vi "DVR Read - CAN Configuration.vi"(11 "Data Value Reference in":refnum<data-value>) -> (3 "CAN Port Configuration":T1 {"Sample Rate (Hz)" format="%#_13g"})   [LabVIEW 2021, in "Performanced XNET CAN Signal Logger.lvlib" / "Performanced XNET CAN Signal Logger.lvclass"]
uses:
  Performanced XNET CAN Signal Logger.lvclass
  Typedef/Def-CAN Port Configuration.ctl
  Performanced XNET CAN Signal Logger.lvclass/Performanced XNET CAN Signal Logger.ctl
  XNET-CAN-Signal-Logger.lvlib
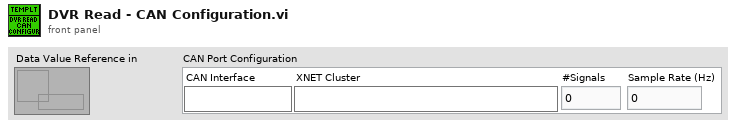
[diagram p1: front panel]
types:
  T1 = typedef "XNET-CAN-Signal-Logger.lvlib/Def-CAN Port Configuration.ctl" = cluster{"CAN Interface":refnum<k21>, "XNET Cluster":refnum<k21>, "#Signals":i32, "Sample Rate (Hz)":dbl}
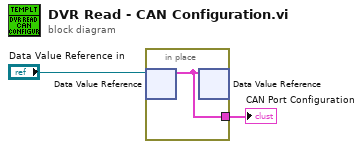
[diagram p0: block diagram]
diagram:
  n1 = in-place {
    in-place-border: [w3] -> w2
    n2 = in-place-dvr #1("Data Value Reference in") -> (w3:T1)  [unwired: 1 out]
    n3 = in-place-dvr #1(w3) -> ()  [unwired: 2 out]
  }
  "CAN Port Configuration" <- w2
